vi "ArmControl.vi"(8 "error in (no error)":errorcluster, 9 "Extension Triggers":cluster{"Retract":dbl, "Extend":dbl}, 10 "Pivot Stick":cluster{"X":dbl, "Y":dbl}, 11 "Wrist Stick":cluster{"X":dbl, "Y":dbl}) -> (0 "error out":errorcluster)   [LabVIEW 2014]
uses:
  Robot Global Data.vi
panel:
  in  "Claw Operation":T1(ring)
  in  "Wrist Multiplier (degrees/sec)":dbl=20.0 format="%#_13g"
  in  "Extend Multiplier (in/sec)":dbl=10.0
  in  "Pivot Multiplier (degrees/sec)":dbl=20.0
  in  "Retract Multiplier (in/sec)":dbl=6.0
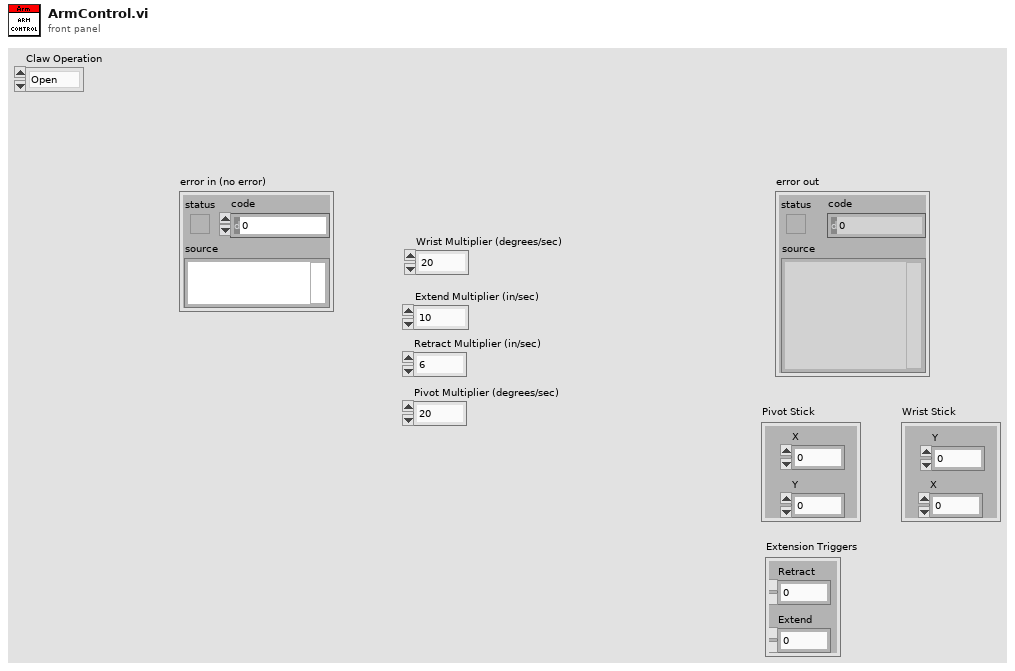
[diagram p1: front panel]
types:
  T1 = enum16{"Open", "Close", "Continue", "Stop", "Toggle"}
  T2 = typedef "WPI_MotorControlDeviceRef.ctl" = cluster{"DeviceStatus":errorcluster, "Type":T3, "PWM":cluster{"Controller":T4, "PWM Channel":T5, "DeadBand":T6}, "CAN":cluster{"Device Number":u8, "Control Mode":T7, "Semaphore":T8, "Max Vout":dbl, "TalonSRX Control Mode":T9}, "Invert":bool, "TransformRef":T10, "InvTransformRef":T10}
  T3 = typedef "WPI_MotorControlType.ctl" = enum16{"PWM", "CAN", "CANTalonSRX"}
  T4 = typedef "FPGA_TypedefDigitalModule.ctl" = enum16{"Controller 1"}
  T5 = typedef "FPGA_DIOPWMChannel.ctl" = enum8{"PWM 0", "PWM 1", "PWM 2", "PWM 3", "PWM 4", "PWM 5", "PWM 6", "PWM 7", "PWM 8", "PWM 9", "PWM MXP 0", "PWM MXP 1", "PWM MXP 2", "PWM MXP 3", "PWM MXP 4", "PWM MXP 5", "PWM MXP 6", "PWM MXP 7", "PWM MXP 8", "PWM MXP 9", "Invalid"}
  T6 = typedef "WPI_PWMDeadband.ctl" = cluster{"Name":string, "maxPositivePwm":i32, "minPositivePwm":i32, "centerPwm":i32, "maxNegativePwm":i32, "minNegativePwm":i32, "angularRange":u16}
  T7 = typedef "WPI_CANJaguar_ControlMode.ctl" = enum8{"Percent VBus", "Current", "Speed", "Position", "Voltage"}
  T8 = typedef "Semaphore RefNum" = refnum<k1>
  T9 = typedef "WPI_CANTalonSRX_APIControlMode.ctl" = enum8{"Percent VBus", "Speed", "Position", "Slave", "Unchanged / Invalid"}
  T10 = typedef "WPI_PWMTransform_ConPane.ctl" = refnum<vi>
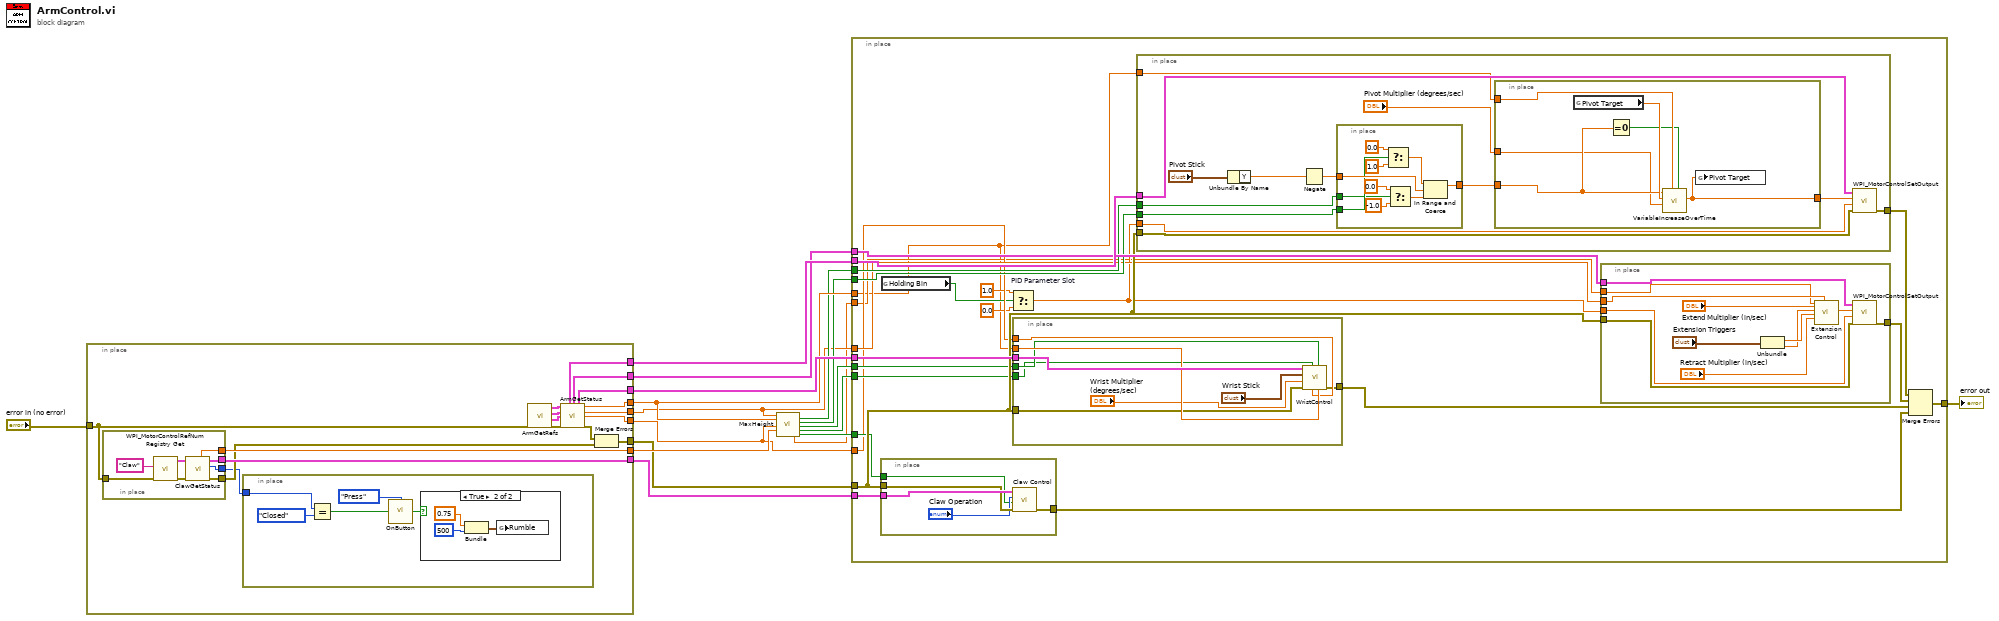
[diagram p0: block diagram]
diagram:
  n1 = in-place {
    in-place-border: "error in (no error)" -> [w22]
    in-place-border: [w25] -> w13
    in-place-border: [w26] -> w15
    in-place-border: [w29] -> w12
    in-place-border: [w24] -> w14
    in-place-border: [w34] -> w11
    in-place-border: [w33] -> w10
    in-place-border: [w32] -> w9
    in-place-border: [w28] -> w2
    in-place-border: [w27] -> w3
    n2 = in-place {
      in-place-border: w22 -> [w49]
      in-place-border: [w46] -> w34
      in-place-border: [w45] -> w33
      in-place-border: [w44] -> w31
      in-place-border: [w43] -> w30
      n3 = call <vilib>:"WPI_MotorControlRefNum Registry Get.vi"("error in (no error)"=w49, "refnum name"="Claw") -> ("error out"=w47:errorcluster, "MotorControlDevRef"=w48:T2)  [unwired: 8 in]
      n4 = call "ClawGetStatus.vi"("error in (no error)"=w47, "MotorControlDevRef"=w48) -> ("error out"=w44:errorcluster, "Claw State"=w43:enum16{"Open", "Closed", "Neither"}, "MotorControlDevRef"=w45:T2, "Claw Angle"=w46:dbl)  [unwired: 5 in, 1 out]
    }
    n5 = in-place {
      in-place-border: w30 -> [w36]
      n6 = Equal?(x=w36, y=enum16{"Open", "Closed", "Neither"}."Closed") -> (x = y?=w37:bool)
      n7 = call "OnButton.vi"("Button"=w37, "Mode"=enum16{"Press", "Release", "Both"}."Press") -> ("Value"=w39:bool)
      n8 = case shown="True" w39 {
        frame False {
        }
        frame True {
          n9 = Bundle("t"=0.75, "f"=i16 500) -> (w42:cluster{"t":dbl, "f":i16})  [unwired: 1 in]
          n10 = global write "Robot Global Data.vi" "Rumble"(w42) -> ()
        }
      }
    }
    n11 = call "ArmGetRefs.vi"("error in (no error)"=w22) -> ("error out"=w21:errorcluster, "Wrist Ref"=w20:T2, "Extension Ref"=w19:T2, "Pivot Ref"=w18:T2)  [unwired: 7 in]
    n12 = call "ArmGetStatus.vi"("Pivot Ref"=w18, "ExtensionRef"=w19, "Wrist Ref"=w20, "error in (no error)"=w21) -> ("Pivot Ref out"=w26:T2, "Extension Ref out"=w25:T2, "Wrist Ref out"=w24:T2, "Pivot angle (rad)"=w29:dbl, "Extension (in.)"=w28:dbl, "Wrist angle (rad, relative to ground)"=w27:dbl, "error out"=w23:errorcluster)  [unwired: 3 in, 2 out]
    n13 = Merge Errors(w23, w31) -> (w32:errorcluster)
  }
  n14 = call "MaxHeight.vi"("Extension Length"=w2, "Pivot Angle"=w12, "Wrist Angle (relative to ground)"=w3, "Claw Angle"=w11) -> ("Max Extension"=w1:dbl, "Disable Pivot Forward"=w6:bool, "Disable Pivot Back"=w7:bool, "Disable Wrist Forward"=w5:bool, "Disable Wrist Back"=w4:bool, "Disable Claw Close"=w8:bool)  [unwired: 9 in, 1 out]
  n15 = in-place {
    in-place-border: [w73] -> w17
    in-place-border: w15 -> [w72]
    in-place-border: w14 -> [w71]
    in-place-border: w13 -> [w70]
    in-place-border: w12 -> [w51]
    in-place-border: w3 -> [w57]
    in-place-border: w10 -> [w69]
    in-place-border: w9 -> [w68]
    in-place-border: w8 -> [w67]
    in-place-border: w7 -> [w66]
    in-place-border: w6 -> [w65]
    in-place-border: w5 -> [w64]
    in-place-border: w4 -> [w63]
    in-place-border: w2 -> [w58]
    in-place-border: w1 -> [w52]
    n16 = in-place {
      in-place-border: w69 -> [w116]
      in-place-border: w67 -> [w112]
      in-place-border: w68 -> [w115]
      in-place-border: [w114] -> w59
      n17 = call "Claw Control.vi"("error in (no error)"=w115, "Disable Claw Close"=w112, "Operation"="Claw Operation", "MotorControlDevRef"=w116) -> ("error out"=w114:errorcluster)  [unwired: 3 in, 2 out]
    }
    n18 = global read "Robot Global Data.vi" "Holding Bin"() -> (w53:bool)
    n19 = Select "PID Parameter Slot"(t=1.0, s=w53, f=0.0) -> (s? t:f=w56:dbl)
    n20 = in-place {
      in-place-border: w71 -> [w82]
      in-place-border: w51 -> [w81]
      in-place-border: w57 -> [w80]
      in-place-border: w68 -> [w79]
      in-place-border: w64 -> [w78]
      in-place-border: w63 -> [w77]
      in-place-border: [w74] -> w62
      n21 = call "WristControl.vi"("Pivot Angle"=w81, "Disable Wrist Forward"=w78, "Wrist Angle (relative to ground)"=w80, "Disable Wrist Back"=w77, "error in (no error)"=w79, "Wrist Multiplier (degrees/second)"="Wrist Multiplier (degrees/sec)", "Wrist Stick"="Wrist Stick", "MotorControlDevRef"=w82) -> ("error out"=w74:errorcluster)  [unwired: 1 in, 2 out]
    }
    n22 = in-place {
      in-place-border: w72 -> [w95]
      in-place-border: w66 -> [w94]
      in-place-border: w65 -> [w93]
      in-place-border: w68 -> [w90]
      in-place-border: [w89] -> w60
      in-place-border: w56 -> [w87]
      in-place-border: w51 -> [w84]
      n23 = Unbundle By Name("Pivot Stick") -> ("Y"=w92:dbl)
      n24 = Negate(x=w92) -> (-x=w91:dbl)
      n25 = in-place {
        in-place-border: w91 -> [w111]
        in-place-border: [w108] -> w86
        in-place-border: w94 -> [w103]
        in-place-border: w93 -> [w102]
        n26 = Select(t=0.0, s=w103, f=1.0) -> (s? t:f=w110:dbl)
        n27 = Select(t=0.0, s=w102, f=-1.0) -> (s? t:f=w109:dbl)
        n28 = In Range and Coerce(upper limit=w110, x=w111, lower limit=w109) -> (coerced(x)=w108:dbl)  [unwired: 1 out]
      }
      n29 = in-place {
        in-place-border: w86 -> [w98]
        in-place-border: [w99] -> w83
        in-place-border: w84 -> [w101]
        in-place-border: "Pivot Multiplier (degrees/sec)" -> [w96]
        n30 = global read "Robot Global Data.vi" "Pivot Target"() -> (w100:dbl)
        n31 = Equal To 0?(x=w98) -> (x = 0?=w97:bool)
        n32 = call "VariableIncreaseOverTime.vi"("Reset to current"=w97, "Current value"=w101, "Multiplier (units/sec)"=w96, "Variable in"=w100, "Joystick input"=w98) -> ("Variable out"=w99:dbl)  [unwired: 6 in]
        n33 = global write "Robot Global Data.vi" "Pivot Target"(w99) -> ()
      }
      n34 = call <vilib>:"WPI_MotorControlSetOutput.vi"("error in (no error)"=w90, "Sync Group / Parameter Slot"=w87, "Output"=w83, "MotorControlDevRef"=w95) -> ("error out"=w89:errorcluster)  [unwired: 5 in, 2 out]
    }
    n35 = in-place {
      in-place-border: w70 -> [w128]
      in-place-border: [w126] -> w61
      in-place-border: w68 -> [w125]
      in-place-border: w58 -> [w123]
      in-place-border: w56 -> [w118]
      in-place-border: w52 -> [w117]
      n36 = Unbundle("Extension Triggers") -> ("Retract"=w122:dbl, "Extend"=w121:dbl)
      n37 = call "Extension Control.vi"("Max Extension"=w117, "Extension Multiplier (in./sec)"="Extend Multiplier (in/sec)", "Extension Trigger"=w121, "Retraction Trigger"=w122, "Retraction Multiplier (in./sec)"="Retract Multiplier (in/sec)", "Extension Position"=w123) -> ("Extension Output"=w124:dbl)  [unwired: 13 in]
      n38 = call <vilib>:"WPI_MotorControlSetOutput.vi"("error in (no error)"=w125, "Sync Group / Parameter Slot"=w118, "Output"=w124, "MotorControlDevRef"=w128) -> ("error out"=w126:errorcluster)  [unwired: 5 in, 2 out]
    }
    n39 = Merge Errors(w60, w61, w62, w59) -> (w73:errorcluster)
  }
  "error out" <- w17
